vi "Convert Module Model to Module Class.vi"(8 "error in":errorcluster, 11 "module model":T1) -> (0 "error out":errorcluster, 3 "module":refnum<class "Module.lvclass">)   [LabVIEW 2020, in "Scan Engine Scripting.lvlib"]
uses:
  Scan Engine Scripting.lvlib
  Modules.lvlibp/RSI Module/Module Models.ctl
  Modules/Module/Module.lvclass
  Scan Engine Dependencies.llb/Error Strings.vi
  Scan Engine Dependencies.llb/Scan Engine Custom Device.lvlib
  Modules.lvlibp/RSI Module/RSI Module.lvclass
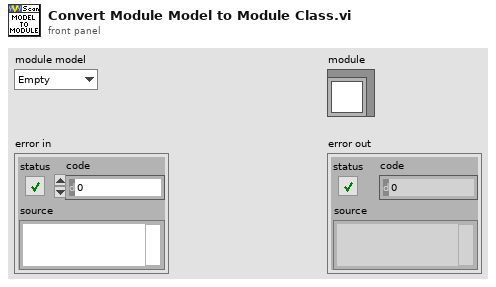
[diagram p1: front panel]
types:
  T1 = typedef "Modules.lvlibp/RSI Module.lvclass/Module Models.ctl" = enum16{"Empty", "NI 9201", "NI 9203", "NI 9205", "NI 9206", "NI 9207", "NI 9208", "NI 9209", "NI 9210", "NI 9211", "NI 9212", "NI 9213", "NI 9214", "NI 9215", "NI 9216", "NI 9217", "NI 9219", "NI 9220", "NI 9221", "NI 9222", "NI 9223", "NI 9224", "NI 9225", "NI 9226", "NI 9227", "NI 9228", "NI 9229", "NI 9233", "NI 9234", "NI 9235", "NI 9236", "NI 9237", "NI 9239", "NI 9242", "NI 9244", "NI 9253", "NI 9263", "NI 9264", "NI 9265", "NI 9266", "NI 9269", "NI 9344", "NI 9350", "NI 9375", "NI 9401", "NI 9402", "NI 9403", "NI 9411", "NI 9421", "NI 9422", "NI 9423", "NI 9425", "NI 9426", "NI 9435", "NI 9436", "NI 9437", "NI 9472", "NI 9474", "NI 9475", "NI 9476", "NI 9477", "NI 9478", "NI 9481", "NI 9482", "NI 9485"}
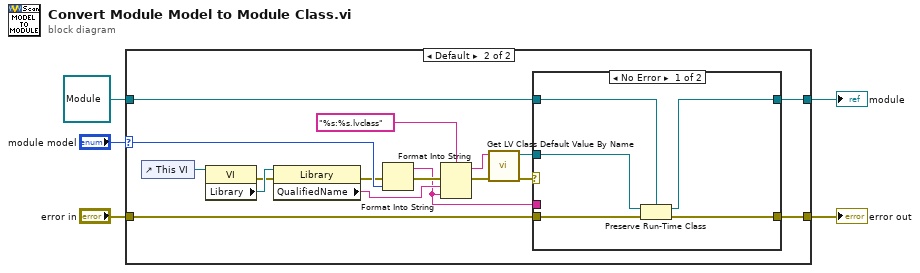
[diagram p0: block diagram]
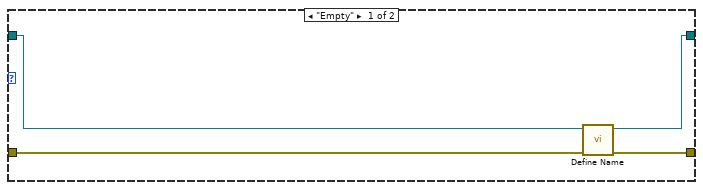
[diagram p2: hidden frame]
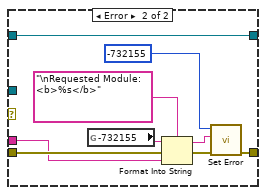
[diagram p3: hidden frame]
diagram:
  n1 = case shown="Default" "module model" {
    selector: "module model" -> [_ w23]
    tunnel: [w9 w20] -> w5
    tunnel: "error in" -> [w7 w26]
    tunnel: [w8 w25] -> w3
    tunnel: refnum<class "Module.lvclass"> refnum ("Scan Engine Scripting.lvlib:Module.lvclass") -> [w6 w19]
    frame "Empty" {
      n2 = call-dynamic "Define Name.vi"("error in"=w7, "module in"=w6) -> ("error out"=w8:errorcluster, "module out"=w9:refnum<class "Module.lvclass">)  [unwired: 8 in]
    }
    frame Default {
      n3 = control-ref of="This VI"() -> (w17:refnum<vi>)
      n4 = property class="VI"(reference=w17) -> (error out=w15:errorcluster, "Library"=w16:refnum<vi>)  [unwired: 1 in, 1 out]
      n5 = property class="Library"(reference=w16, error in=w15) -> (error out=w14:errorcluster, "QualifiedName"=w13:string)  [unwired: 1 out]
      n6 = Format Into String(error in=w14, w23) -> (resulting string=w10:string, error out=w24:errorcluster)  [unwired: 2 in]
      n7 = Format Into String(format string="%s:%s.lvclass", error in=w24, w13, w10) -> (resulting string=w11:string, error out=w18:errorcluster)  [unwired: 1 in]
      n8 = call <vilib>:"Get LV Class Default Value By Name.vi"("error in (no error)"=w18, "class name"=w11) -> ("error out"=w22:errorcluster, "object"=w21:refnum<class>)  [unwired: 8 in]
      n9 = case shown="No Error" w22 {
        tunnel: [w28 w37] -> w20
        tunnel: w26 -> [w31 w40]
        tunnel: [w30 w39] -> w25
        tunnel: w21 -> [w29 _]
        tunnel: w19 -> [w27 w37]
        tunnel: w10 -> [_ w32]
        frame No Error {
          n10 = Preserve Run-Time Class(object in=w29, error in=w31, 2:w27) -> (object out=w28:refnum<class "Module.lvclass">, error out=w30:errorcluster)
        }
        frame Error {
          n11 = global read "Error Strings.vi" "-732155"() -> (w35:string)
          n12 = Format Into String(format string="\nRequested Module: <b>%s</b>", initial string=w35, error in=w40, w32) -> (resulting string=w34:string, error out=w36:errorcluster)
          n13 = call "Set Error.vi"("error in (no error)"=w36, "Message"=w34, "Code"=-732155) -> ("error out"=w39:errorcluster)  [unwired: 8 in]
        }
      }
    }
  }
  "module" <- w5
  "error out" <- w3
